vi "ExecuteClimb.vi"(8 "Error In":errorcluster, 10 "Left Climb":T1={"DeviceStatus"={"status"=FALSE, "code"=0, "source"=""}, "Type"=enum."PWM", "PWM"={"PWM Channel"=enum."PWM 1", "DeadBand"={"Name"="", "maxPositivePwm"=0, "minPositivePwm"=0, "centerPwm"=0, "maxNegativePwm"=0, "minNegativePwm"=0, "angularRange"=0}}, "CAN"={"Device Number"=0, "SetOutput VI Ref"=variant(enum8{"Percent VBus", "Current", "Speed", "Position", "Voltage"} enum."Percent VBus"), "GetOutput VI Ref"=variant(refnum<k1> refnum), "Enable VI Ref"=variant(dbl 12.0), "Disable VI Ref"=variant(enum8{"Percent VBus", "Speed", "Position", "Slave", "Unchanged / Invalid", "Voltage Compensation", "Current", "Motion Profile"} enum."Percent VBus"), "Data"=variant}, "Invert"=FALSE, "DIO PWM"={"PWM \"Enable\" Channel"=enum."Invalid", "DIOChannel"=enum."Invalid", "PWM Rate"=0.0}}, 11 "Right Climb":T1={"DeviceStatus"={"status"=FALSE, "code"=0, "source"=""}, "Type"=enum."PWM", "PWM"={"PWM Channel"=enum."PWM 1", "DeadBand"={"Name"="", "maxPositivePwm"=0, "minPositivePwm"=0, "centerPwm"=0, "maxNegativePwm"=0, "minNegativePwm"=0, "angularRange"=0}}, "CAN"={"Device Number"=0, "SetOutput VI Ref"=variant(enum8{"Percent VBus", "Current", "Speed", "Position", "Voltage"} enum."Percent VBus"), "GetOutput VI Ref"=variant(refnum<k1> refnum), "Enable VI Ref"=variant(dbl 12.0), "Disable VI Ref"=variant(enum8{"Percent VBus", "Speed", "Position", "Slave", "Unchanged / Invalid", "Voltage Compensation", "Current", "Motion Profile"} enum."Percent VBus"), "Data"=variant}, "Invert"=FALSE, "DIO PWM"={"PWM \"Enable\" Channel"=enum."Invalid", "DIOChannel"=enum."Invalid", "PWM Rate"=0.0}}) -> (0 "Error Out":errorcluster)   [LabVIEW 2020]
uses:
  <vilib>/Rock Robotics/WPI/MotorControl/WPI_MotorControlDeviceRef.ctl
  <vilib>/Rock Robotics/WPI/MotorControl/WPI_MotorControlType.ctl
  <vilib>/Rock Robotics/SystemInterfaces/DIO/FPGA_DIOPWMChannel.ctl
  <vilib>/Rock Robotics/WPI/PWM/WPI_PWMDeadband.ctl
  <vilib>/Rock Robotics/SystemInterfaces/DIO/FPGA_DIOChannel.ctl
  <vilib>/Rock Robotics/WPI/Solenoid/WPI_SolenoidValue.ctl
  ClimbGlobals.vi
  <vilib>/Rock Robotics/WPI/Solenoid/WPI_SolenoidSetEnum.vi
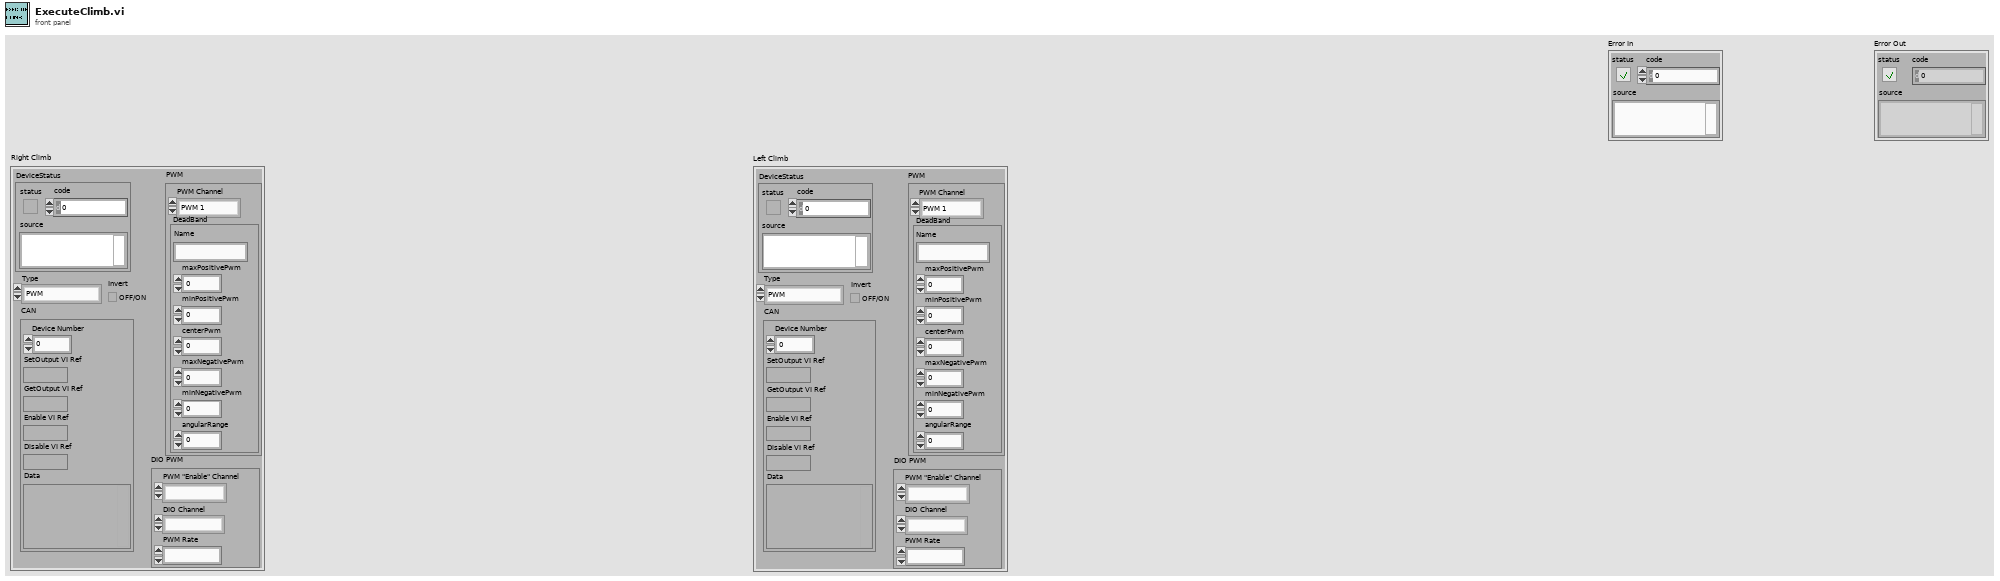
[diagram p1: front panel]
types:
  T1 = typedef "WPI_MotorControlDeviceRef.ctl" = cluster{"DeviceStatus":errorcluster, "Type":T2, "PWM":cluster{"PWM Channel":T3, "DeadBand":T4}, "CAN":cluster{"Device Number":u8, "SetOutput VI Ref":variant, "GetOutput VI Ref":variant, "Enable VI Ref":variant, "Disable VI Ref":variant, "Data":variant}, "Invert":bool, "DIO PWM":cluster{"PWM \"Enable\" Channel":T3, "DIOChannel":T5, "PWM Rate":dbl}}
  T2 = typedef "WPI_MotorControlType.ctl" = enum16{"PWM", "CAN", "DIO PWM"}
  T3 = typedef "FPGA_DIOPWMChannel.ctl" = enum8{"PWM 0", "PWM 1", "PWM 2", "PWM 3", "PWM 4", "PWM 5", "PWM 6", "PWM 7", "PWM 8", "PWM 9", "PWM MXP 0", "PWM MXP 1", "PWM MXP 2", "PWM MXP 3", "PWM MXP 4", "PWM MXP 5", "PWM MXP 6", "PWM MXP 7", "PWM MXP 8", "PWM MXP 9", "Invalid"}
  T4 = typedef "WPI_PWMDeadband.ctl" = cluster{"Name":string, "maxPositivePwm":i32, "minPositivePwm":i32, "centerPwm":i32, "maxNegativePwm":i32, "minNegativePwm":i32, "angularRange":u16}
  T5 = typedef "FPGA_DIOChannel.ctl" = enum8{"DIO 0", "DIO 1", "DIO 2", "DIO 3", "DIO 4", "DIO 5", "DIO 6", "DIO 7", "DIO 8", "DIO 9", "DIO MXP 0", "DIO MXP 1", "DIO MXP 2", "DIO MXP 3", "DIO MXP 4", "DIO MXP 5", "DIO MXP 6", "DIO MXP 7", "DIO MXP 8", "DIO MXP 9", "DIO MXP 10", "DIO MXP 11", "DIO MXP 12", "DIO MXP 13", "DIO MXP 14", "DIO MXP 15", "SPI Port CS1", "SPI Port CS2", "SPI Port CS3", "SPI Port MISO", "SPI Port MOSI", "Invalid"}
  T6 = typedef "WPI_SolenoidValue.ctl" = enum16{"Off", "On", "Forward", "Reverse"}
  T7 = typedef "WPI_SolenoidDevRef.ctl" = cluster{"DevStatus":errorcluster, "Pneumatics Control Module":u8, "Forward Solenoid Channel":T8, "Reverse Solenoid Channel":T8}
  T8 = typedef "WPI_SolenoidChannel.ctl" = enum8{"Solenoid 0", "Solenoid 1", "Solenoid 2", "Solenoid 3", "Solenoid 4", "Solenoid 5", "Solenoid 6", "Solenoid 7", "Solenoid 8", "Solenoid 9", "Solenoid 10", "Solenoid 11", "Solenoid 12", "Solenoid 13", "Solenoid 14", "Solenoid 15", "Invalid"}
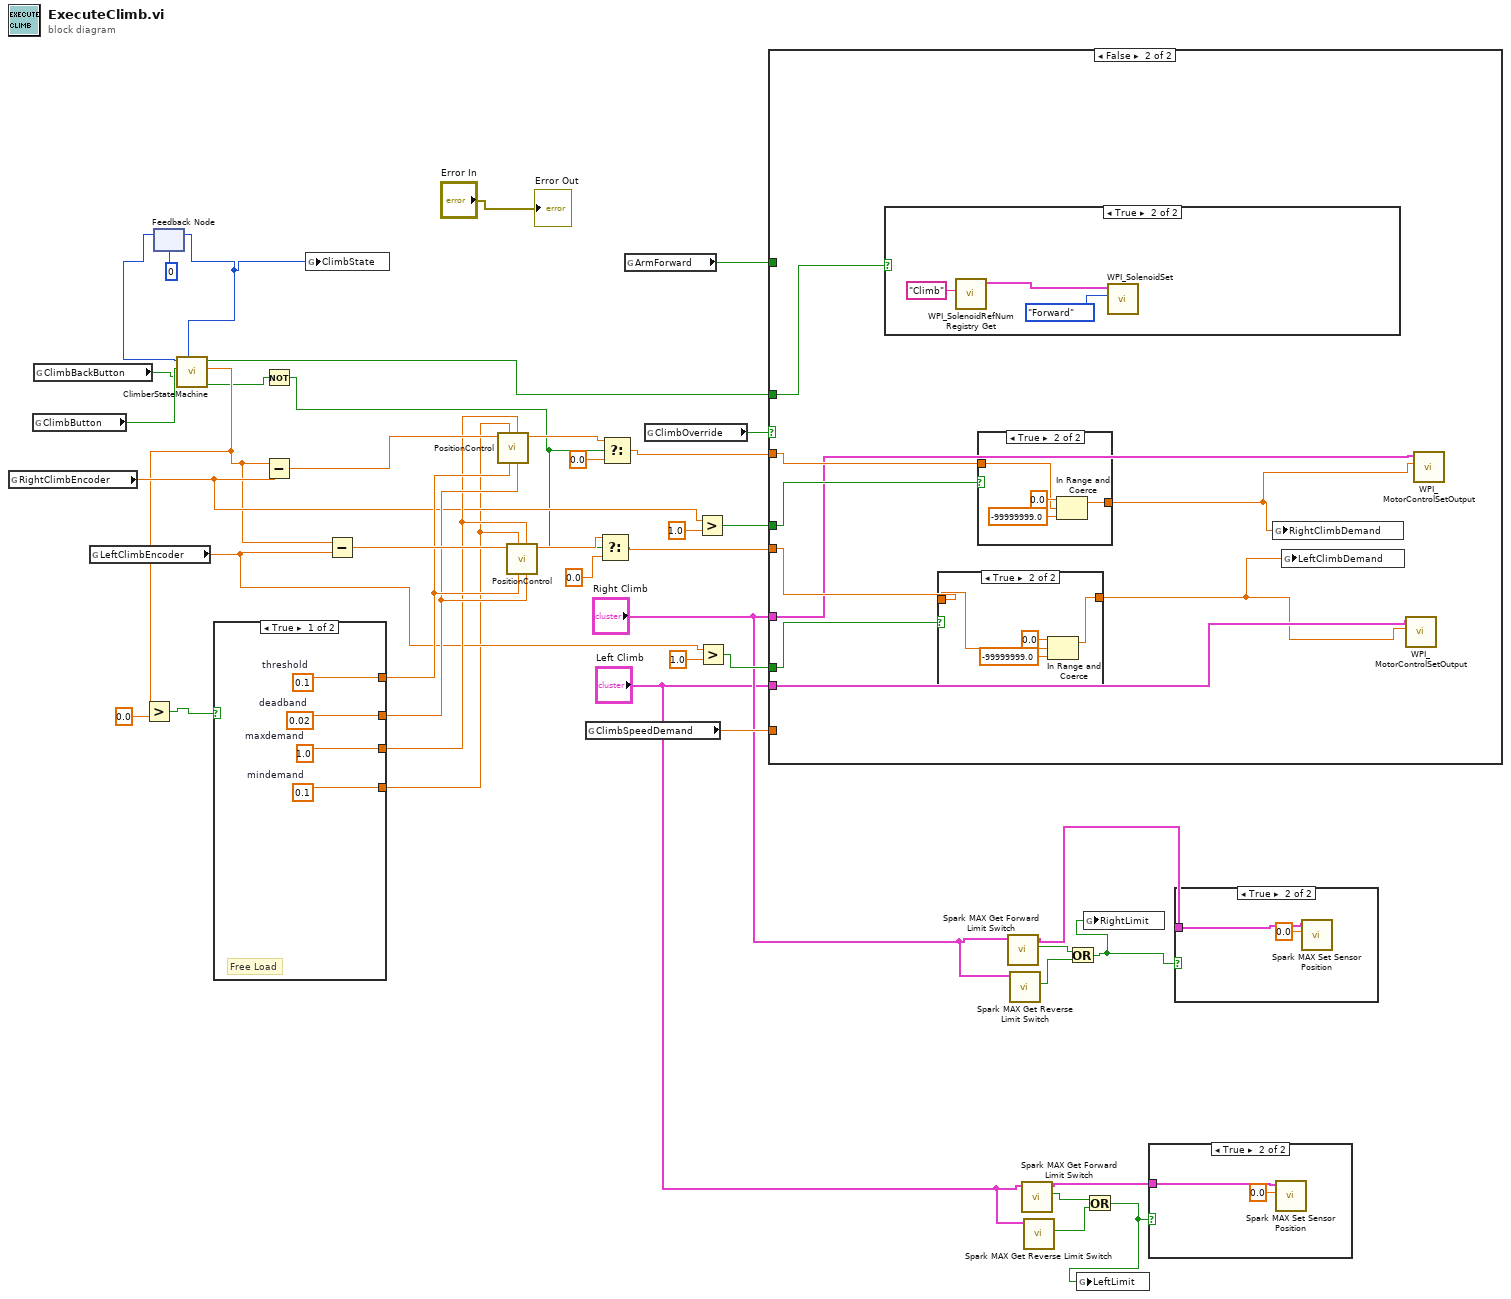
[diagram p0: block diagram]
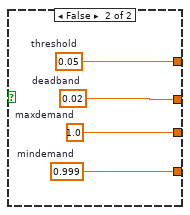
[diagram p4: hidden frame]
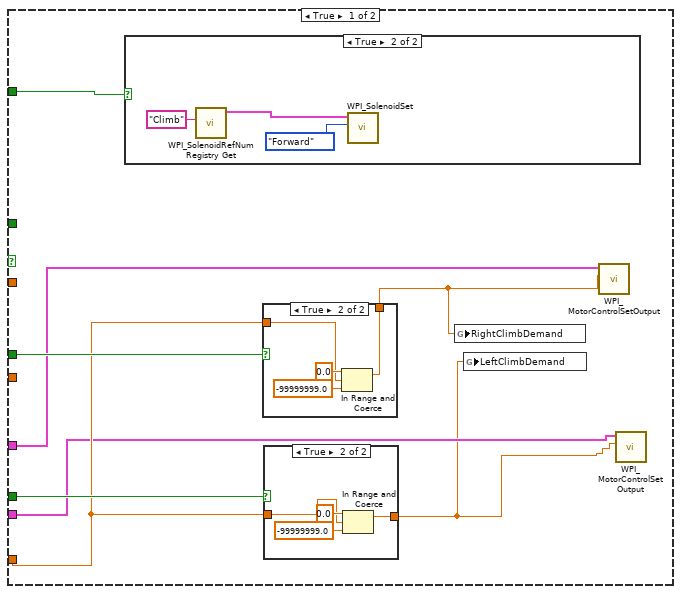
[diagram p5: hidden frame]
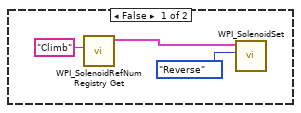
[diagram p8: hidden frame]
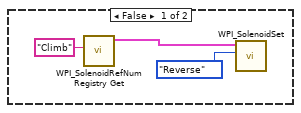
[diagram p11: hidden frame]
diagram:
  n1 = global read "ClimbGlobals.vi" "RightClimbEncoder"() -> (w24:dbl)
  n2 = global read "ClimbGlobals.vi" "ClimbButton"() -> (w41:bool)
  n3 = global read "ClimbGlobals.vi" "ClimbBackButton"() -> (w22:bool)
  n4 = global read "ClimbGlobals.vi" "LeftClimbEncoder"() -> (w25:dbl)
  n5 = feedback #1(0 ("NextState")) -> (w43:i32)
  n6 = call "ClimberStateMachine.vi"("CimbBackButton"=w22, "ClimbButton"=w41, "State"=w43) -> ("DisablePosCon"=w12:bool, "ArmPosition"=w20:dbl, "ArmForward"=w32:bool, "NextState"=w40:i32)  [unwired: 5 in]
  n7 = Greater?(x=w20, y=0.0) -> (0:w19:bool)
  n8 = feedback-in #1(w40) -> ()
  n9 = case shown="True" w19 {
    tunnel: [w44 w51] -> w36
    tunnel: [w45 w50] -> w35
    tunnel: [w46 w49] -> w34
    tunnel: [w47 w48] -> w23
    frame True {
      w44 = 0.1  # threshold
      w45 = 0.02  # deadband
      w46 = 1.0  # maxdemand
      w47 = 0.1  # mindemand
      # "Free Load"
    }
    frame False {
      w51 = 0.05  # threshold
      w50 = 0.02  # deadband
      w48 = 0.999  # mindemand
      w49 = 1.0  # maxdemand
    }
  }
  n10 = Not(x=w12) -> (.not. x?=w11:bool)
  n11 = Subtract(x=w20, y=w24) -> (x-y=w38:dbl)
  n12 = global write "ClimbGlobals.vi" "ClimbState"(w40) -> ()
  n13 = Subtract(x=w20, y=w25) -> (x-y=w37:dbl)
  n14 = call "PositionControl.vi"("deadband"=w35, "maxdemand"=w34, "threshold"=w36, "mindemand"=w23, "Error"=w38) -> ("output variable"=w17:dbl)  [unwired: 5 in, 1 out]
  n15 = call "PositionControl.vi"("deadband"=w35, "maxdemand"=w34, "threshold"=w36, "mindemand"=w23, "Error"=w37) -> ("output variable"=w15:dbl)  [unwired: 5 in, 1 out]
  n16 = global read "ClimbGlobals.vi" "ClimbSpeedDemand"() -> (w33:dbl)
  n17 = Select(t=w15, s=w11, f=0.0) -> (s? t:f=w16:dbl)
  n18 = Select(t=w17, s=w11, f=0.0) -> (s? t:f=w18:dbl)
  n19 = global read "ClimbGlobals.vi" "ArmForward"() -> (w39:bool)
  n20 = global read "ClimbGlobals.vi" "ClimbOverride"() -> (w30:bool)
  n21 = Greater?(x=w24, y=1.0) -> (0:w27:bool)
  n22 = Greater?(x=w25, y=1.0) -> (0:w26:bool)
  n23 = case shown="False" w30 {
    tunnel: "Right Climb" -> [w55 w78]
    tunnel: "Left Climb" -> [w54 w79]
    tunnel: w39 -> [w59 _]
    tunnel: w33 -> [w56 _]
    tunnel: w32 -> [_ w84]
    tunnel: w18 -> [_ w80]
    tunnel: w16 -> [_ w81]
    tunnel: w27 -> [w58 w83]
    tunnel: w26 -> [w57 w82]
    frame True {
      n24 = case shown="True" w59 {
        frame False {
          n25 = call <vilib>:"WPI_SolenoidRefNum Registry Get.vi"("refnum name"="Climb") -> ("SolenoidDevRef"=w71:T7)  [unwired: 9 in, 1 out]
          n26 = call-poly <vilib>:"WPI_SolenoidSet.vi"("Value"=WPI_SolenoidValue."Reverse", "SolenoidDevRef"=w71) -> ()  [unwired: 8 in, 2 out]
        }
        frame True {
          n27 = call <vilib>:"WPI_SolenoidRefNum Registry Get.vi"("refnum name"="Climb") -> ("SolenoidDevRef"=w74:T7)  [unwired: 9 in, 1 out]
          n28 = call-poly <vilib>:"WPI_SolenoidSet.vi"("Value"=WPI_SolenoidValue."Forward", "SolenoidDevRef"=w74) -> ()  [unwired: 8 in, 2 out]
        }
      }
      n29 = case shown="True" w58 {
        tunnel: w56 -> [w65 w67]
        tunnel: [w65 w66] -> w52
        frame False {
        }
        frame True {
          n30 = In Range and Coerce(upper limit=0.0, x=w67, lower limit=-99999999.0) -> (coerced(x)=w66:dbl)  [unwired: 1 out]
        }
      }
      n31 = case shown="True" w57 {
        tunnel: w56 -> [w60 w62]
        tunnel: [w60 w61] -> w53
        frame False {
        }
        frame True {
          n32 = In Range and Coerce(upper limit=0.0, x=w62, lower limit=-99999999.0) -> (coerced(x)=w61:dbl)  [unwired: 1 out]
        }
      }
      n33 = global write "ClimbGlobals.vi" "RightClimbDemand"(w52) -> ()
      n34 = global write "ClimbGlobals.vi" "LeftClimbDemand"(w53) -> ()
      n35 = call <vilib>:"WPI_MotorControlSetOutput.vi"("Output"=w52, "MotorControlDevRef"=w55) -> ()  [unwired: 7 in, 3 out]
      n36 = call <vilib>:"WPI_MotorControlSetOutput.vi"("Output"=w53, "MotorControlDevRef"=w54) -> ()  [unwired: 7 in, 3 out]
    }
    frame False {
      n37 = case shown="True" w84 {
        frame False {
          n38 = call <vilib>:"WPI_SolenoidRefNum Registry Get.vi"("refnum name"="Climb") -> ("SolenoidDevRef"=w96:T7)  [unwired: 9 in, 1 out]
          n39 = call-poly <vilib>:"WPI_SolenoidSet.vi"("Value"=WPI_SolenoidValue."Reverse", "SolenoidDevRef"=w96) -> ()  [unwired: 8 in, 2 out]
        }
        frame True {
          n40 = call <vilib>:"WPI_SolenoidRefNum Registry Get.vi"("refnum name"="Climb") -> ("SolenoidDevRef"=w99:T7)  [unwired: 9 in, 1 out]
          n41 = call-poly <vilib>:"WPI_SolenoidSet.vi"("Value"=WPI_SolenoidValue."Forward", "SolenoidDevRef"=w99) -> ()  [unwired: 8 in, 2 out]
        }
      }
      n42 = case shown="True" w82 {
        tunnel: [w90 w92] -> w76
        tunnel: w81 -> [w90 w91]
        frame False {
        }
        frame True {
          n43 = In Range and Coerce(upper limit=0.0, x=w91, lower limit=-99999999.0) -> (coerced(x)=w92:dbl)  [unwired: 1 out]
        }
      }
      n44 = case shown="True" w83 {
        tunnel: w80 -> [w85 w87]
        tunnel: [w85 w86] -> w77
        frame False {
        }
        frame True {
          n45 = In Range and Coerce(upper limit=0.0, x=w87, lower limit=-99999999.0) -> (coerced(x)=w86:dbl)  [unwired: 1 out]
        }
      }
      n46 = global write "ClimbGlobals.vi" "RightClimbDemand"(w77) -> ()
      n47 = global write "ClimbGlobals.vi" "LeftClimbDemand"(w76) -> ()
      n48 = call <vilib>:"WPI_MotorControlSetOutput.vi"("Output"=w76, "MotorControlDevRef"=w79) -> ()  [unwired: 7 in, 3 out]
      n49 = call <vilib>:"WPI_MotorControlSetOutput.vi"("Output"=w77, "MotorControlDevRef"=w78) -> ()  [unwired: 7 in, 3 out]
    }
  }
  n50 = call <vilib>:"Spark MAX Get Forward Limit Switch.vi"("MotorControlDevRef in"="Right Climb") -> ("Hard Limit Fwd"=w8:bool, "MotorControlDevRef out"=w7:T1)  [unwired: 7 in, 2 out]
  n51 = call <vilib>:"Spark MAX Get Reverse Limit Switch.vi"("MotorControlDevRef in"="Right Climb") -> ("Hard Limit Rev"=w9:bool)  [unwired: 7 in, 3 out]
  n52 = call <vilib>:"Spark MAX Get Forward Limit Switch.vi"("MotorControlDevRef in"="Left Climb") -> ("Hard Limit Fwd"=w4:bool, "MotorControlDevRef out"=w6:T1)  [unwired: 7 in, 2 out]
  n53 = call <vilib>:"Spark MAX Get Reverse Limit Switch.vi"("MotorControlDevRef in"="Left Climb") -> ("Hard Limit Rev"=w3:bool)  [unwired: 7 in, 3 out]
  n54 = Or(x=w8, y=w9) -> (x .or. y?=w2:bool)
  n55 = global write "ClimbGlobals.vi" "RightLimit"(w2) -> ()
  n56 = Or(x=w4, y=w3) -> (x .or. y?=w1:bool)
  n57 = global write "ClimbGlobals.vi" "LeftLimit"(w1) -> ()
  n58 = case shown="True" w1 {
    tunnel: w6 -> [_ w102]
    frame False {
    }
    frame True {
      n59 = call <vilib>:"Spark MAX Set Sensor Position.vi"("Position"=0.0, "MotorControlDeviceRef"=w102) -> ()  [unwired: 8 in, 2 out]
    }
  }
  n60 = case shown="True" w2 {
    tunnel: w7 -> [_ w104]
    frame False {
    }
    frame True {
      n61 = call <vilib>:"Spark MAX Set Sensor Position.vi"("Position"=0.0, "MotorControlDeviceRef"=w104) -> ()  [unwired: 8 in, 2 out]
    }
  }
  "Error Out" <- "Error In"
